vi "konfiguracjaDanychLINX.vi"(8 "Error In":errorcluster, 9 "Kierunki":bool[](array[boolean]), 10 "Wybór komory":T1, 11 "LINX Resource":T2) -> (0 "Error Out":errorcluster, 3 "LINX Out":T2)   [LabVIEW 2014]
uses:
  <vilib>/MakerHub/LINX/Private/Type Defs/LINX Ref.ctl
  <vilib>/MakerHub/LINX/Private/Type Defs/Platform.ctl
  <vilib>/MakerHub/LINX/Private/Type Defs/Interface.ctl
  <vilib>/MakerHub/LINX/Private/Device/Type Defs/LINX Device Config.ctl
  <vilib>/MakerHub/LINX/Private/Device/Type Defs/TCP Config.ctl
  <vilib>/MakerHub/LINX/Private/Device/Type Defs/Channels.ctl
  parametryKomorVIs/WyborKomory.ctl
  AkcjaGFV.ctl
  <vilib>/MakerHub/LINX/Public/Peripherals/Digital/Digital Write N Chans.vi
  <vilib>/MakerHub/LINX/Private/Local IO/LinxDigitalWrite.vi
  <vilib>/MakerHub/LINX/Public/Utilities/Check Channel.vi
  <vilib>/MakerHub/LINX/Private/Utilties/Generate Error.vi
  <vilib>/MakerHub/LINX/LMH-LINX.lvlib
  <vilib>/MakerHub/LINX/Private/Device/Device.lvlib
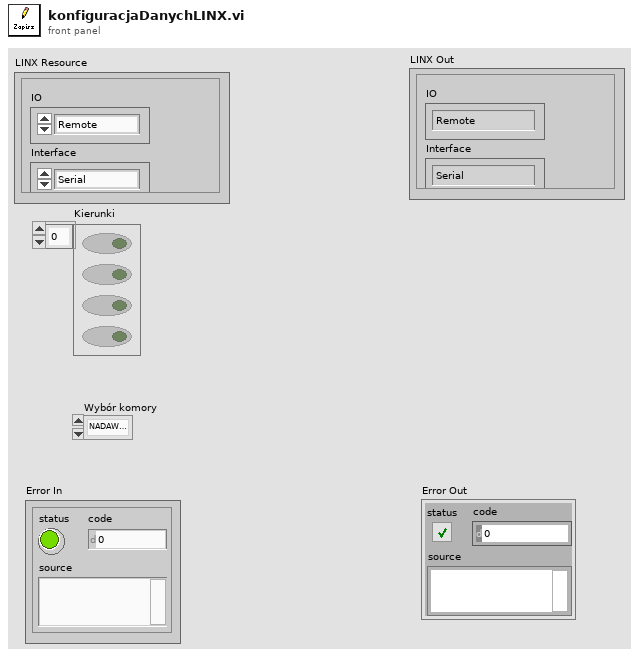
[diagram p1: front panel]
types:
  T1 = typedef "WyborKomory.ctl" = enum16{"NADAWCZA", "ODBIORCZA"}
  T2 = typedef "LMH-LINX.lvlib/LINX Ref.ctl" = cluster{"IO":T3, "Interface":T4, "LINX Device Config":T5}
  T3 = typedef "LMH-LINX.lvlib/Platform.ctl" = enum16{"Remote", "Local"}
  T4 = typedef "LMH-LINX.lvlib/Interface.ctl" = enum16{"Serial", "TCP"}
  T5 = typedef "LMH-LINX.lvlib/Device.lvlib/LINX Device Config.ctl" = cluster{"Interface":T4, "COM Port":refnum<visa-resource-name>, "TCP Configuration":T6, "Device Family":u8, "Device ID":u8, "Device Name":string, "TCP Ref":refnum<k5>, "Channels":T7}
  T6 = typedef "LMH-LINX.lvlib/Device.lvlib/TCP Config.ctl" = cluster{"IP Address":string, "Port":u16}
  T7 = typedef "LMH-LINX.lvlib/Channels.ctl" = cluster{"DI":u8[], "DO":u8[], "AI":u8[], "AO":u8[], "PWM":u8[], "QE":u8[], "UART":u8[], "I2C 2":u8[], "SPI":u8[], "CAN":u8[], "Servo":u8[], "AI Ref (V)":dbl, "AI Resolution (Bits)":u8, "AO Ref (V)":dbl, "AO Resolution (Bits)":u8}
  T8 = typedef "AkcjaGFV.ctl" = enum16{"Czytaj", "Zapisz", "Reset"}
  T9 = typedef "PinoutLista.ctl" = cluster{"LEWO":u8, "PRAWO":u8, "GÓRA":u8, "Dӣ":u8, "CZUJNIK":u8, "I2C ADRES":u8}
  T10 = cluster{"Kierunki[0]":bool, "Kierunki[1]":bool, "Kierunki[2]":bool, "Kierunki[3]":bool, "Kierunki[4]":bool, "Kierunki[5]":bool, "Kierunki[6]":bool, "Kierunki[7]":bool, "Kierunki[8]":bool}
  T11 = typedef "WyjsciaParametry.ctl" = cluster{"Nad. lewo":bool, "Nad.  prawo":bool, "Nad.  gora":bool, "Nad. do³":bool, "Dzialanie":bool, "Pomiar":bool, "Odb. lewo":bool, "Odb.  prawo":bool, "Odb.  gora":bool, "Odb. dol":bool, "Pozostalo punktow":i32, "Nad. elewacja":i32, "Nad. azymut":i32, "Odb. elewacja":i32, "Odb. azymut":i32, "TCP Error":bool, "TCP Error Code":i32, "LINX Error":bool, "LINX Error Code":i32}
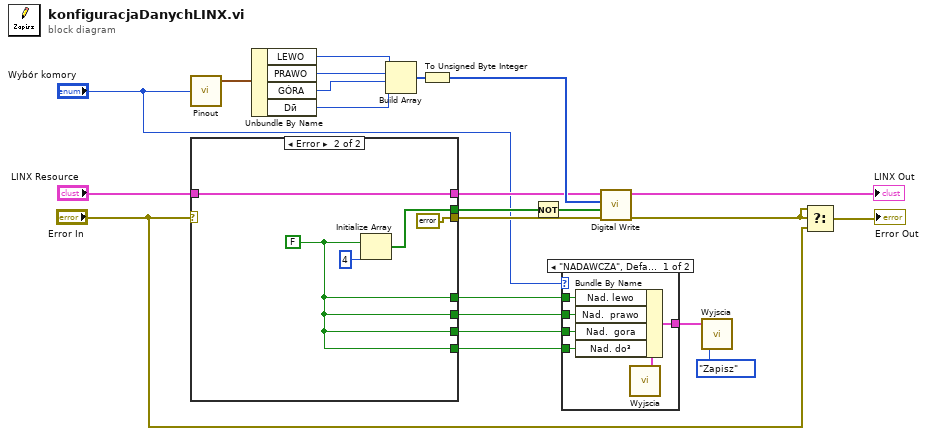
[diagram p0: block diagram]
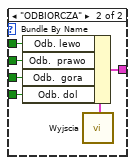
[diagram p2: hidden frame]
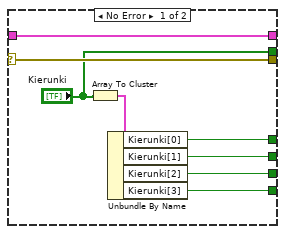
[diagram p3: hidden frame]
diagram:
  n1 = call "Pinout.vi"("Wybór komory"="Wybór komory") -> ("Wyjœcie"=w21:T9)  [unwired: 4 in]
  n2 = case shown="Error" "Error In" {
    selector: "Error In" -> [w31 _]
    tunnel: ["Kierunki" w34] -> w22
    tunnel: [w30 w36] -> w13
    tunnel: [w31 errorcluster {"status"=FALSE, "code"=0, "source"=""} ("error IO")] -> w12
    tunnel: "LINX Resource" -> [w30 w36]
    tunnel: [w27 w32] -> w5
    tunnel: [w26 w32] -> w4
    tunnel: [w25 w32] -> w3
    tunnel: [w24 w32] -> w2
    frame No Error {
      n3 = Array To Cluster(array="Kierunki") -> (cluster=w28:T10)
      n4 = Unbundle By Name(w28) -> ("Kierunki[0]"=w27:bool, "Kierunki[1]"=w26:bool, "Kierunki[2]"=w25:bool, "Kierunki[3]"=w24:bool)
    }
    frame Error {
      w32 = FALSE
      n5 = Initialize Array(w32, 4 ("dimension size")) -> (w34:bool[])
    }
  }
  n6 = Unbundle By Name(w21) -> ("LEWO"=w17:u8, "PRAWO"=w16:u8, "GÓRA"=w15:u8, "Dӣ"=w14:u8)
  n7 = Build Array(w17, w16, w15, w14) -> (w20:u8[])
  n8 = To Unsigned Byte Integer(number=w20) -> (unsigned 8bit integer=w18:u8[])
  n9 = Not(x=w22) -> (.not. x?=w19:bool[])
  n10 = case shown="\"NADAWCZA\", Default" "Wybór komory" {
    tunnel: [w42 w48] -> w6
    tunnel: w2 -> [w41 w47]
    tunnel: w3 -> [w40 w46]
    tunnel: w5 -> [w38 w45]
    tunnel: w4 -> [w39 w44]
    frame "NADAWCZA", Default {
      n11 = call "Wyjscia.vi"() -> ("Wyjœcie"=w37:T11)  [unwired: 5 in]
      n12 = Bundle By Name(cluster=w37, "Nad. lewo"=w38, "Nad.  prawo"=w39, "Nad.  gora"=w40, "Nad. do³"=w41) -> (w42:T11)
    }
    frame "ODBIORCZA" {
      n13 = call "Wyjscia.vi"() -> ("Wyjœcie"=w43:T11)  [unwired: 5 in]
      n14 = Bundle By Name(cluster=w43, "Odb. lewo"=w45, "Odb.  prawo"=w44, "Odb.  gora"=w46, "Odb. dol"=w47) -> (w48:T11)
    }
  }
  n15 = call-poly <vilib>:"Digital Write.vi"("Error In"=w12, "Values"=w19, "DO Channels"=w18, "LINX Resource"=w13) -> ("Error Out"=w10:errorcluster, "LINX Resource"=→"LINX Out":T2)  [unwired: 6 in]
  n16 = call "Wyjscia.vi"("Akcja"=AkcjaGFV."Zapisz", "Wejœcie"=w6) -> ()  [unwired: 3 in, 1 out]
  n17 = Select(t=w10, s=w10, f="Error In") -> (s? t:f=→"Error Out":errorcluster)
